vi "AWG Output.vi"(6 "Channel Name (1)":u16(ring)=1 items=["1"=1, "2"=2, "3"=3, "4"=4], 8 "error in (no error)":errorcluster, 10 "Enable Output (T: Enable)":bool=TRUE, 11 "VISA resource name":refnum<visa-resource-name>="GPIB0::1::INSTR") -> (0 "error out":errorcluster)   [LabVIEW 2021]
uses:
  <instrlib>/Tektronix AWG 5000 7000 Series/Tektronix AWG 5000 7000 Series.lvlib
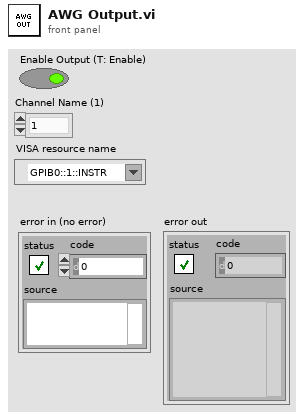
[diagram p1: front panel]
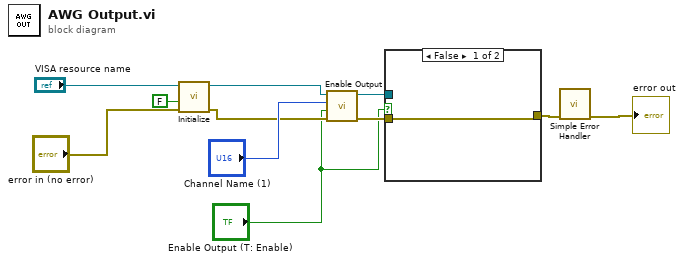
[diagram p0: block diagram]
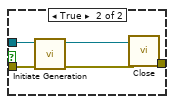
[diagram p2: hidden frame]
diagram:
  n1 = call <instrlib>:"Initialize.vi"("error in (no error)"="error in (no error)", "Reset (False)"=FALSE ("Reset? (F: No)"), "VISA resource name"="VISA resource name") -> ("error out"=w2:errorcluster, "VISA resource name out"=w3:refnum<visa-resource-name>)  [unwired: 7 in]
  n2 = call <instrlib>:"Enable Output.vi"("error in (no error)"=w2, "Enable Output (T: Enable)"="Enable Output (T: Enable)", "Channel Name (1)"="Channel Name (1)", "VISA resource name"=w3) -> ("error out"=w6:errorcluster, "VISA resource name out"=w5:refnum<visa-resource-name>)  [unwired: 6 in]
  n3 = case shown="False" "Enable Output (T: Enable)" {
    tunnel: [w12 w17] -> w8
    tunnel: w6 -> [w12 w16]
    tunnel: w5 -> [_ w15]
    frame False {
    }
    frame True {
      n4 = call <instrlib>:"Initiate Generation.vi"("error in (no error)"=w16, "VISA resource name"=w15) -> ("error out"=w13:errorcluster, "VISA resource name out"=w14:refnum<visa-resource-name>)  [unwired: 8 in]
      n5 = call <instrlib>:"Close.vi"("error in (no error)"=w13, "VISA resource name"=w14) -> ("error out"=w17:errorcluster)  [unwired: 9 in]
    }
  }
  n6 = call <vilib>:"Simple Error Handler.vi"("error in (no error)"=w8) -> ("error out"=→"error out":errorcluster)  [unwired: 4 in, 4 out]
